vi "ReportPath.vi"(11 "s":bool) -> (0 "error out":errorcluster, 3 "created path":path)   [LabVIEW 2013]
uses:
  Control/Buffer.vi
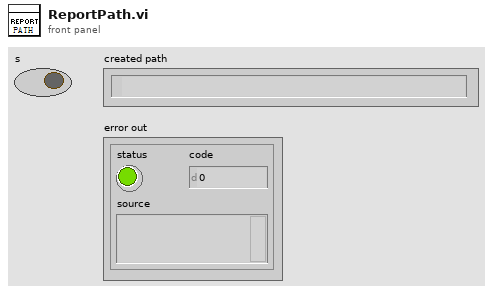
[diagram p1: front panel]
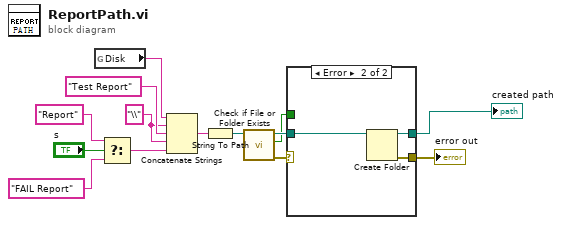
[diagram p0: block diagram]
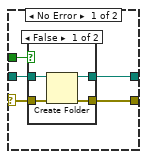
[diagram p2: hidden frame]
diagram:
  w2 = "\\" ("string")
  n1 = global read "Buffer.vi" "Disk"() -> (w1:string)
  n2 = Select(t="Report" ("string"), s="s", f="FAIL Report" ("string")) -> (s? t:f=w10:string)
  n3 = Concatenate Strings(w1, w2, "Test Report" ("string"), w2, w10) -> (w4:string)
  n4 = String To Path(string=w4) -> (path=w8:path)
  n5 = call <vilib>:"Check if File or Folder Exists.vi"("path"=w8) -> ("error out"=w5:errorcluster, "file or folder exists?"=w6:bool, "dup path"=w7:path)  [unwired: 8 in]
  n6 = case shown="Error" w5 {
    selector: w5 -> [w16 _]
    tunnel: w7 -> [w19 w28]
    tunnel: w6 -> [w18 _]
    tunnel: [w17 w27] -> w9
    tunnel: [w15 w26] -> w14
    frame No Error {
      n7 = case shown="False" w18 {
        tunnel: w19 -> [w23 w25]
        tunnel: [w22 w25] -> w17
        tunnel: w16 -> [w21 w24]
        tunnel: [w20 w24] -> w15
        frame False {
          n8 = Create Folder(path (use dialog)=w23, error in=w21) -> (created path=w22:path, error out=w20:errorcluster)  [unwired: 1 in, 1 out]
        }
        frame True {
        }
      }
    }
    frame Error {
      n9 = Create Folder(path (use dialog)=w28) -> (created path=w27:path, error out=w26:errorcluster)  [unwired: 2 in, 1 out]
    }
  }
  "error out" <- w14
  "created path" <- w9
